vi "Bad Setting Error.vi"(7 "vi name":string, 8 "error in (no error)":errorcluster, 10 "value":string, 11 "key":string) -> (0 "error out":errorcluster)   [LabVIEW 2017, in "PXImc.lvlib" / "PXImc Transceiver.lvclass"]
uses:
  PXImc Transceiver.lvclass
  Errors.ctl
  <vilib>/NI/Memory Manager/Static Errors.lvlib
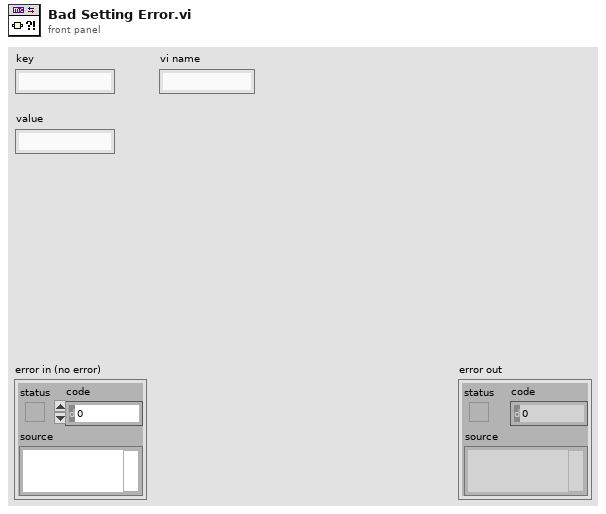
[diagram p1: front panel]
types:
  T1 = typedef "PXImc.lvlib/PXImc Transceiver.lvclass/Errors.ctl" = enum8{"Bad Setting", "Duplicate Stream ID"}
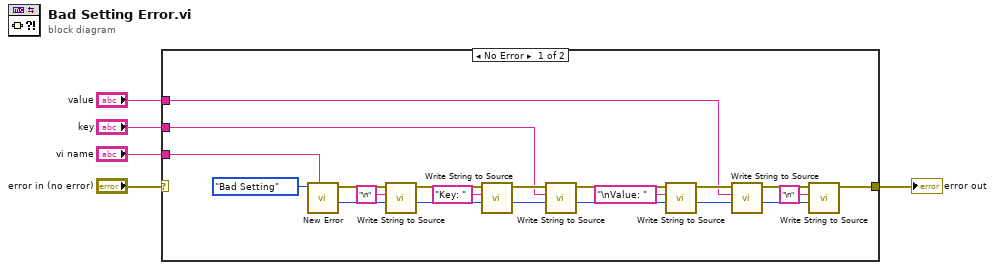
[diagram p0: block diagram]
diagram:
  n1 = case shown="No Error" "error in (no error)" {
    selector: "error in (no error)" -> [_ w27]
    tunnel: [w17 w27] -> w4
    tunnel: "vi name" -> [w25 _]
    tunnel: "value" -> [w9 _]
    tunnel: "key" -> [w14 _]
    frame No Error {
      n2 = call "New Error.vi"("vi name"=w25, "error"=Errors."Bad Setting") -> ("initial offset"=w6:i32, "error"=w24:errorcluster)  [unwired: 8 in]
      n3 = call <vilib>:"Write String to Source.vi"("offset"=w6, "string"="\n", "error in"=w24) -> ("new offset"=w22:i32, "error out"=w21:errorcluster)  [unwired: 7 in]
      n4 = call <vilib>:"Write String to Source.vi"("offset"=w22, "string"="Key: ", "error in"=w21) -> ("new offset"=w15:i32, "error out"=w16:errorcluster)  [unwired: 7 in]
      n5 = call <vilib>:"Write String to Source.vi"("offset"=w15, "string"=w14, "error in"=w16) -> ("new offset"=w13:i32, "error out"=w12:errorcluster)  [unwired: 7 in]
      n6 = call <vilib>:"Write String to Source.vi"("offset"=w13, "string"="\nValue: ", "error in"=w12) -> ("new offset"=w10:i32, "error out"=w11:errorcluster)  [unwired: 7 in]
      n7 = call <vilib>:"Write String to Source.vi"("offset"=w10, "string"=w9, "error in"=w11) -> ("new offset"=w7:i32, "error out"=w8:errorcluster)  [unwired: 7 in]
      n8 = call <vilib>:"Write String to Source.vi"("offset"=w7, "string"="\n", "error in"=w8) -> ("error out"=w17:errorcluster)  [unwired: 7 in, 1 out]
    }
    frame Error {
    }
  }
  "error out" <- w4
